vi "ReadFile.vi"(8 "error in (no error)":errorcluster, 11 "ROFile in":refnum<class "ROFile.lvclass">) -> (0 "error out":errorcluster, 2 "data":i32[](array[numeric]))   [LabVIEW 2021, in "ROFile.lvclass"]
uses:
  ROFile.lvclass
  ROFile.lvclass/ROFile.ctl
  File/File.lvclass
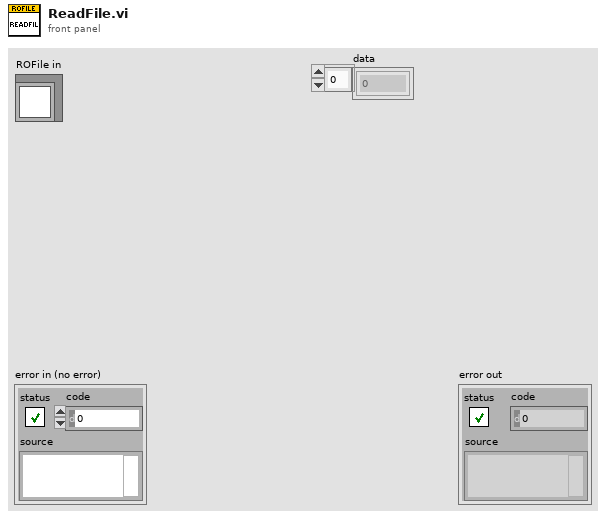
[diagram p1: front panel]
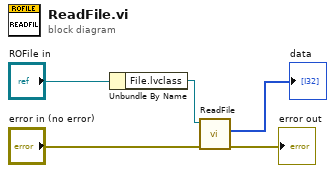
[diagram p0: block diagram]
diagram:
  n1 = Unbundle By Name("ROFile in") -> ("File.lvclass"=w1:refnum<class "File.lvclass">)
  n2 = call "ReadFile.vi"("error in (no error)"="error in (no error)", "File in"=w1) -> ("error out"=→"error out":errorcluster, "data"=→"data":i32[])  [unwired: 8 in]
